vi "AdaptToInputs.vi"(3 "Term Types":T1, 4 "XRef":refnum<vi>, 5 "State In":T5) -> (0 "Reply":string[](array[string]), 2 "State Out":T5)   [LabVIEW 2012, in "OpenG Delete Elements from Array.xnode"]
uses:
  OpenG Delete Elements from Array.xnode
  State.ctl
  <vilib>/XNodeSupport/XNodeTermTypeIDPairs.ctl
  <vilib>/XNodeSupport/XNodeTermTypeIDPair.ctl
  <vilib>/XNodeSupport/XNodeType.ctl
  <vilib>/XNodeSupport/XNodeString.ctl
  <userlib>/_LAVAcr/Scripting Tools/XNode Support/TypeDefs/Array Dimension Tests.ctl
  <userlib>/_LAVAcr/Scripting Tools/XNode Support/Find term type by ID_type.vi
  <userlib>/_LAVAcr/Scripting Tools/XNode Support/XNode Support.lvlib
  <vilib>/XNodeSupport/NI_XNodeSupport.lvlib
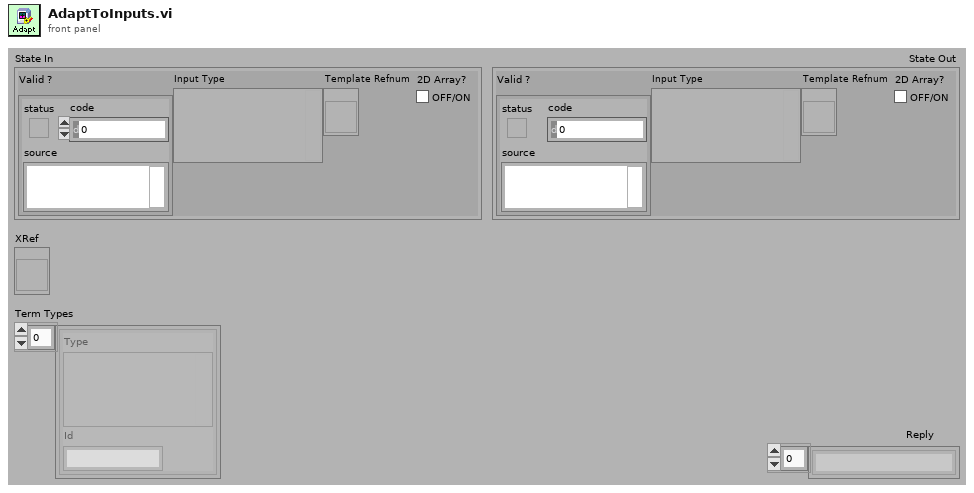
[diagram p1: front panel]
types:
  T1 = typedef "NI_XNodeSupport.lvlib/XNodeTermTypeIDPairs.ctl" = T2[]
  T2 = typedef "NI_XNodeSupport.lvlib/XNodeTermTypeIDPair.ctl" = cluster{"Type":T3, "Id":T4}
  T3 = typedef "NI_XNodeSupport.lvlib/XNodeType.ctl" = variant
  T4 = typedef "NI_XNodeSupport.lvlib/XNodeString.ctl" = string
  T5 = typedef "OpenG Delete Elements from Array.xnode/State.ctl" = cluster{"Valid ?":errorcluster, "Input Type":variant, "Template Refnum":refnum<vi>, "2D Array?":bool}
  T6 = typedef "Scripting Tools.lvlib/XNode Support.lvlib/Array Dimension Tests.ctl" = enum16{"No Check", "At Least n dimensions", "Exactly N Dimensions", "No More Than N Dimensions"}
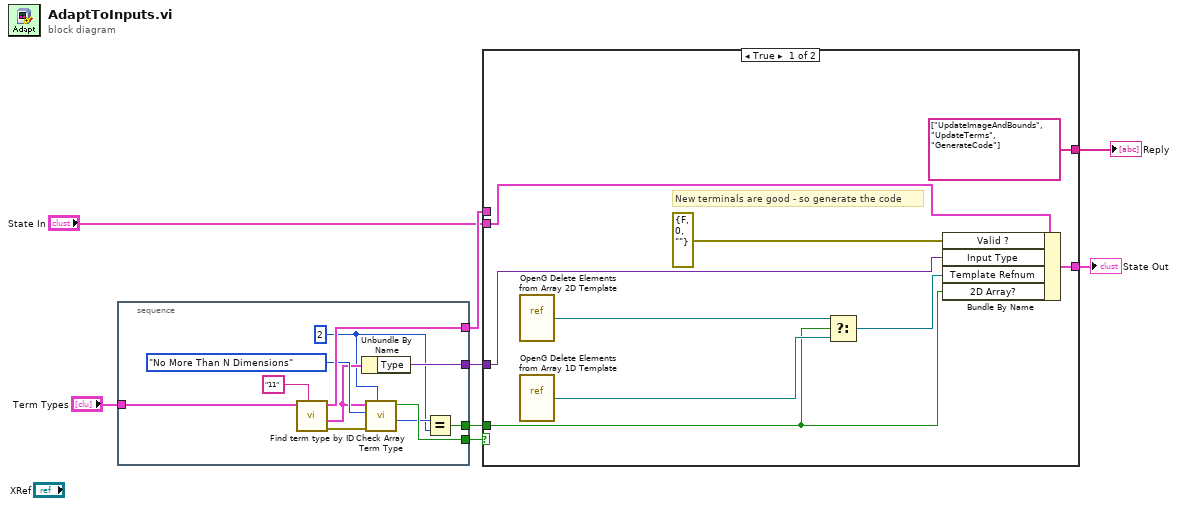
[diagram p0: block diagram]
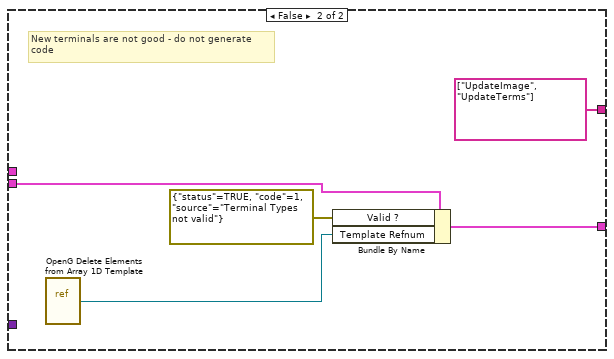
[diagram p2: hidden frame]
diagram:
  n1 = stacked-sequence {
    tunnel: "Term Types" -> [w19]
    tunnel: [w18] -> w7
    tunnel: [w12] -> w8
    tunnel: [w13] -> w6
    tunnel: [w9] -> w5
    frame #0 {
      w10 = 2 ("Dimensions Required")
      n2 = call-poly <userlib>:"Find term type by ID.vi"("Search ID"="11", "Term Types"=w19) -> ("error out"=w16:errorcluster, "Term Type"=w14:T2, "Other Term Types"=w18:T2[])  [unwired: 1 in, 6 out]
      n3 = Unbundle By Name(w14) -> ("Type"=w13:T3)
      n4 = call <userlib>:"Check Array Term Type.vi"("Dimensions Required"=w10, "error in (no error)"=w16, "Dimension Check"=Array_Dimension_Tests."No More Than N Dimensions", "Term Type"=w14) -> ("Array Dimensions"=w11:i32, "Is Good ?"=w12:bool)  [unwired: 1 in, 5 out]
      n5 = Equal?(x=w11, y=w10) -> (x = y?=w9:bool)
    }
  }
  n6 = case shown="True" w8 {
    tunnel: w7 -> [_ _]
    tunnel: "State In" -> [w28 w33]
    tunnel: [w26 w31] -> w1
    tunnel: [string[] ["UpdateImageAndBounds", "UpdateTerms", "GenerateCode"] ("Reply") string[] ["UpdateImage", "UpdateTerms"] ("Reply")] -> w2
    tunnel: w6 -> [w25 _]
    tunnel: w5 -> [w21 _]
    frame True {
      # "New terminals are good - so generate the code"
      n7 = vi-ref "OpenG Delete Elements from Array 2D Template.vi"() -> (w24:refnum<vi>)
      n8 = vi-ref "OpenG Delete Elements from Array 1D Template.vi"() -> (w23:refnum<vi>)
      n9 = Select(t=w24, s=w21, f=w23) -> (s? t:f=w22:refnum<vi>)
      n10 = Bundle By Name(cluster=w28, "Valid ?"=errorcluster {"status"=FALSE, "code"=0, "source"=""}, "Input Type"=w25, "Template Refnum"=w22, "2D Array?"=w21) -> (w26:T5)
    }
    frame False {
      # "New terminals are not good - do not generate\ncode"
      n11 = vi-ref "OpenG Delete Elements from Array 1D Template.vi"() -> (w29:refnum<vi>)
      n12 = Bundle By Name(cluster=w33, "Valid ?"=errorcluster {"status"=TRUE, "code"=1, "source"="Terminal Types not valid"}, "Template Refnum"=w29) -> (w31:T5)
    }
  }
  "Reply" <- w2
  "State Out" <- w1
